vi "Benchmark mupExpr_parse_and_eval.vi"(8 "error in (no error)":errorcluster, 10 "Iterations":i32, 11 "Expression":string) -> (0 "error out":errorcluster, 2 "x":dbl[](array[numeric]), 3 "y":dbl[](array[numeric]), 5 "dt average":dbl)   [LabVIEW 2015]
uses:
  mupExpr/mupExpr.lvclass/mupExpr.ctl
  mupExpr/Eval.vi
  mupLib/mupSetVarValue.vi
  mupLib/mupEval.vi
  mupLib/mupCheckError.vi
  mupLib/mupLibPath.vi
  <vilib>/Utility/error.llb/Error Cluster From Error Code.vi
  mupExpr/mupExpr.lvclass
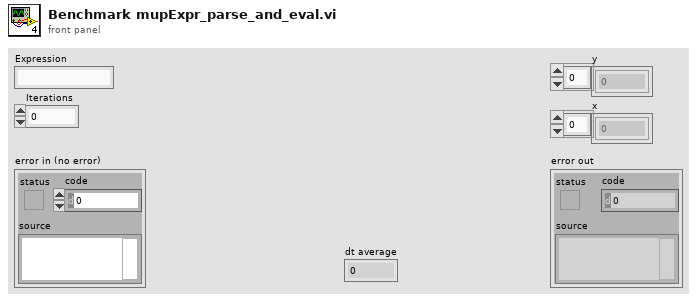
[diagram p1: front panel]
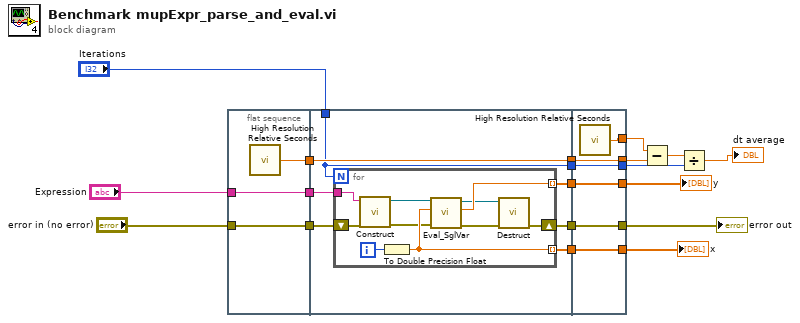
[diagram p0: block diagram]
diagram:
  n1 = flat-sequence {
    tunnel: "error in (no error)" -> [w22]
    tunnel: [w22] -> w17
    tunnel: [w21] -> w12
    tunnel: [w20] -> w4
    tunnel: "Expression" -> [w20]
    tunnel: w17 -> [w29]
    tunnel: [w28] -> w16
    tunnel: [w27] -> w15
    tunnel: [w26] -> w14
    tunnel: [w25] -> w13
    tunnel: w12 -> [w25]
    tunnel: "Iterations" -> [w24]
    tunnel: [w24] -> w6
    tunnel: w4 -> [w23]
    tunnel: [w43] -> w18
    tunnel: [w44] -> w19
    tunnel: [w45] -> w1
    tunnel: w16 -> [w45]
    tunnel: w15 -> [w44]
    tunnel: w14 -> [w43]
    tunnel: [w42] -> w10
    tunnel: w13 -> [w42]
    tunnel: [w41] -> w11
    tunnel: [w40] -> w7
    tunnel: w6 -> [w40]
    frame #0 {
      n2 = call <vilib>:"High Resolution Relative Seconds.vi"() -> ("relative seconds"=w21:dbl)
    }
    frame #1 {
      n3 = for {
        N: w24 -> [_]
        shift-right: [w30] -> w28
        shift-left: w29 -> [w33]
        tunnel: [w37] -> w27 mode=indexing
        tunnel: [w38] -> w26 mode=indexing
        tunnel: w23 -> [w36]
        i -> [w39]
        n4 = call "Construct.vi"("error in (no error)"=w33, "Expression"=w36) -> ("error out"=w34:errorcluster, "muExpr out"=w35:refnum<class "mupExpr.lvclass">)  [unwired: 7 in, 1 out]
        n5 = To Double Precision Float(number=w39) -> (double precision float=w38:dbl)
        n6 = call "Eval_SglVar.vi"("error in (no error)"=w34, "varValue"=w38, "muExpr in"=w35) -> ("error out"=w32:errorcluster, "Result"=w37:dbl, "muExpr out"=w31:refnum<class "mupExpr.lvclass">)  [unwired: 6 in]
        n7 = call "Destruct.vi"("error in (no error)"=w32, "muExpr in"=w31) -> ("error out"=w30:errorcluster)  [unwired: 9 in]
      }
    }
    frame #2 {
      n8 = call <vilib>:"High Resolution Relative Seconds.vi"() -> ("relative seconds"=w41:dbl)
    }
  }
  n9 = Subtract(x=w11, y=w10) -> (x-y=w8:dbl)
  n10 = Divide(x=w8, y=w7) -> (x/y=→"dt average":dbl)
  "y" <- w19
  "x" <- w18
  "error out" <- w1
